vi "Set Log File Additional Properties.vi"(8 "error in":errorcluster, 9 "property values":string[](array[string]), 10 "property names":string[](array[string]), 11 "log file in":T1 format="%.0x") -> (0 "error out":errorcluster, 3 "log file out":T1 format="%.0x")   [LabVIEW 2027, in "Embedded Data Logger Scripting.lvlib"]
uses:
  Embedded Data Logger Scripting.lvlib
  <vilib>/NI VeriStand/Custom Device API/Custom Device Item Ref.ctl
  Shared/Constants.vi
  <vilib>/NI VeriStand/Custom Device API/Set Item Property (String Array).vi
  <vilib>/NI VeriStand/Custom Device API/Custom Device API.lvlib
  Shared/Embedded Data Logger Shared.lvlib
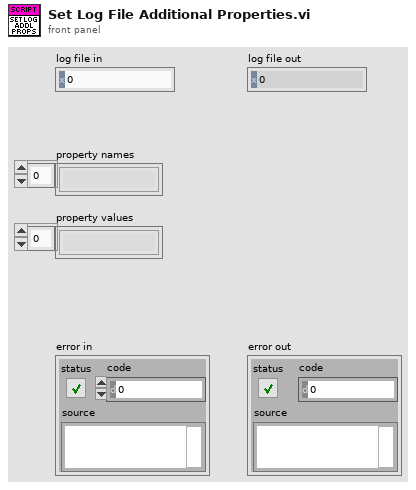
[diagram p1: front panel]
types:
  T1 = typedef "Custom Device API.lvlib/Custom Device Item Ref.ctl" = u64
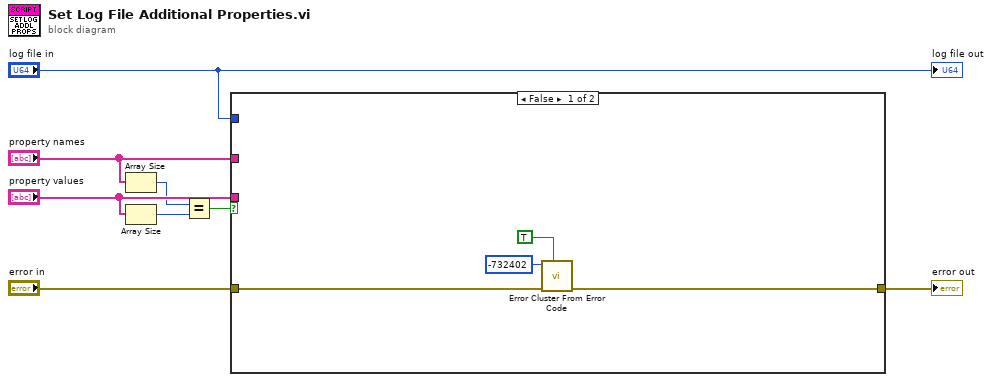
[diagram p0: block diagram]
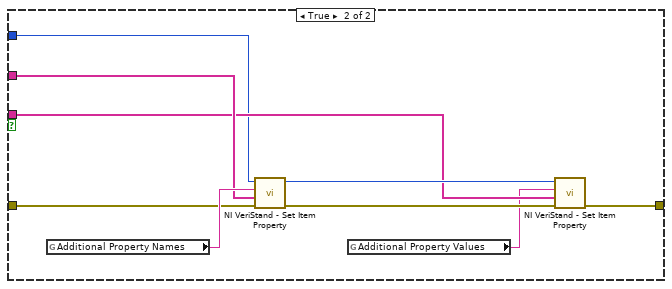
[diagram p2: hidden frame]
diagram:
  n1 = Array Size(array="property names") -> (size(s)=w2:i32)
  n2 = Array Size(array="property values") -> (size(s)=w3:i32)
  n3 = Equal?(x=w2, y=w3) -> (x = y?=w1:bool)
  n4 = case shown="False" w1 {
    tunnel: "error in" -> [w12 w20]
    tunnel: "property names" -> [_ w19]
    tunnel: [w11 w17] -> w7
    tunnel: "property values" -> [_ w15]
    tunnel: "log file in" -> [_ w13]
    frame False {
      n5 = call <vilib>:"Error Cluster From Error Code.vi"("show call chain? (False)"=TRUE, "error in (no error)"=w12, "error code (0)"=-732402) -> ("error out"=w11:errorcluster)  [unwired: 6 in]
    }
    frame True {
      n6 = global read "Constants.vi" "Additional Property Names"() -> (w21:string)
      n7 = call-poly <vilib>:"NI VeriStand - Set Item Property.vi"("error in (no error)"=w20, "Value"=w19, "Property Name"=w21, "Item Ref in"=w13) -> ("error out"=w18:errorcluster, "Item Ref out"=w16:T1)  [unwired: 6 out]
      n8 = global read "Constants.vi" "Additional Property Values"() -> (w14:string)
      n9 = call-poly <vilib>:"NI VeriStand - Set Item Property.vi"("error in (no error)"=w18, "Value"=w15, "Property Name"=w14, "Item Ref in"=w16) -> ("error out"=w17:errorcluster)  [unwired: 7 out]
    }
  }
  "error out" <- w7
  "log file out" <- "log file in"
